vi "Scale Vertical Range.vi"(8 "error in (no error)":errorcluster, 11 "TAS/TPC Config In":T1={"Vertical Range (V)"=0.2, "Vertical Offset (0.0 divs)"=0.0, "Bandwidth"=0, "Probe Attenuation (10.0)"=1.0, "Vertical Coupling"=1, "Impedance"=0, "Multiplication factor"=1.0, "Channel"=enum."None"} {"Impedance" items=["1M", "75", "50"]; "Vertical Coupling" items=["AC", "DC", "Ground"]; "Bandwidth" items=["FULL", "250 MHz", "150 MHz", "20 MHz"]}) -> (0 "error out":errorcluster, 3 "TAS/TPC Config Out":T1={"Vertical Range (V)"=0.2, "Vertical Offset (0.0 divs)"=0.0, "Bandwidth"=0, "Probe Attenuation (10.0)"=1.0, "Vertical Coupling"=1, "Impedance"=0, "Multiplication factor"=1.0, "Channel"=enum."None"} {"Impedance" items=["1M", "75", "50"]; "Vertical Coupling" items=["AC", "DC", "Ground"]; "Bandwidth" items=["FULL", "250 MHz", "150 MHz", "20 MHz"]})   [LabVIEW 2017, in "Scope.lvlib"]
uses:
  Scope.lvlib
  Controls/TPC.ctl
  Controls/Channels.ctl
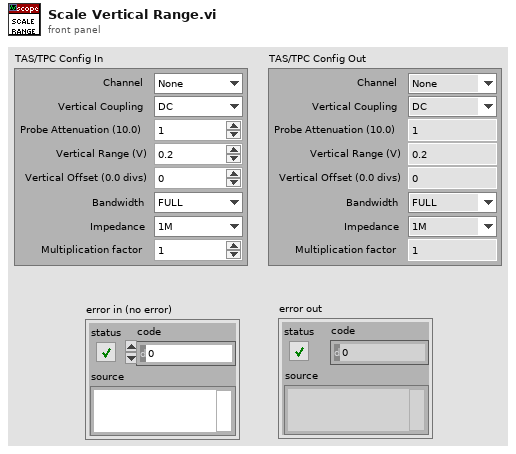
[diagram p1: front panel]
types:
  T1 = typedef "Scope.lvlib/TPC.ctl" = cluster{"Vertical Range (V)":dbl, "Vertical Offset (0.0 divs)":dbl, "Bandwidth":i32, "Probe Attenuation (10.0)":dbl, "Vertical Coupling":u16, "Impedance":u16, "Multiplication factor":dbl, "Channel":T2}
  T2 = typedef "Scope.lvlib/Channels.ctl" = enum16{"Channel 1", "Channel 2", "Channel 3", "Channel 4", "Math", "Reference A", "Reference B", "Reference C", "Reference D", "B1", "B2", "None"}
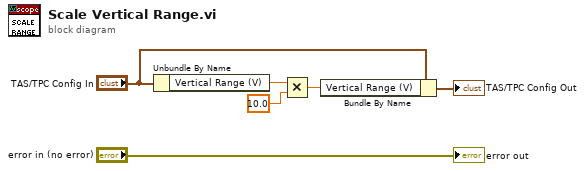
[diagram p0: block diagram]
diagram:
  n1 = Unbundle By Name("TAS/TPC Config In") -> ("Vertical Range (V)"=w6:dbl)
  n2 = Multiply(x=w6, y=10.0) -> (x*y=w3:dbl)
  n3 = Bundle By Name(cluster="TAS/TPC Config In", "Vertical Range (V)"=w3) -> (→"TAS/TPC Config Out":T1)
  "error out" <- "error in (no error)"
